vi "test Add and Get Timing Channels.vi"(8 "error in":errorcluster, 11 "TestCase in":refnum<class "Scripting.lvclass">) -> (0 "error out":errorcluster)   [LabVIEW 2024, in "Scripting.lvclass"]
uses:
  Scripting.lvclass
  <vilib>/NI VeriStand/Custom Device API/Custom Device Item Ref.ctl
  Scripting.lvclass/Scripting.ctl
  <vilib>/addons/_JKI Toolkits/VI Tester/TestCase.llb/TestCase.lvclass
  Scripting/AIM/AIM ARINC 429 Scripting.lvlib
  <vilib>/NI VeriStand/Custom Device API/Custom Device API.lvlib
  C:/Program Files/National Instruments/LabVIEW 2024/vi.lib/addons/_JKI Toolkits/VI Tester/TestCase.llb/TestCase.lvclass
panel:
  out "TestCase out":refnum<class "Scripting.lvclass">
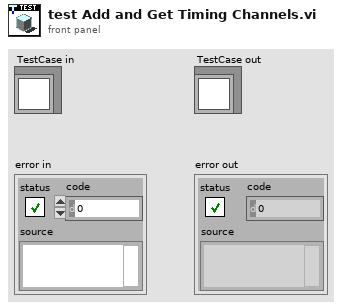
[diagram p1: front panel]
types:
  T1 = typedef "Custom Device API.lvlib/Custom Device Item Ref.ctl" = u64
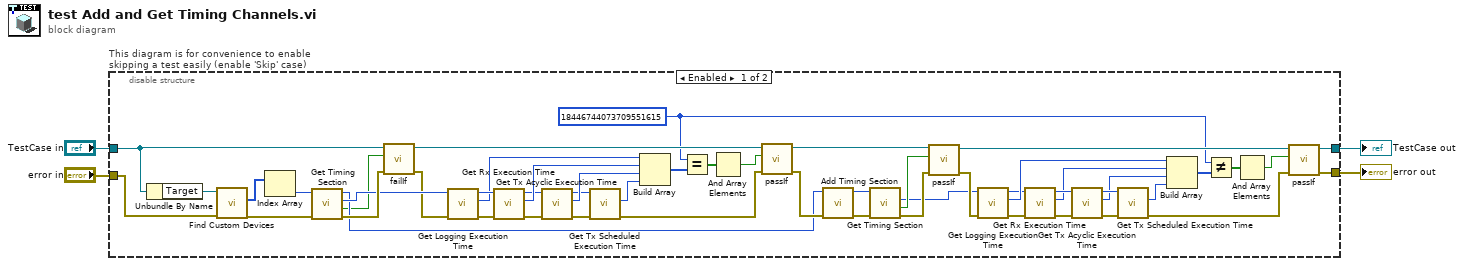
[diagram p0: block diagram]
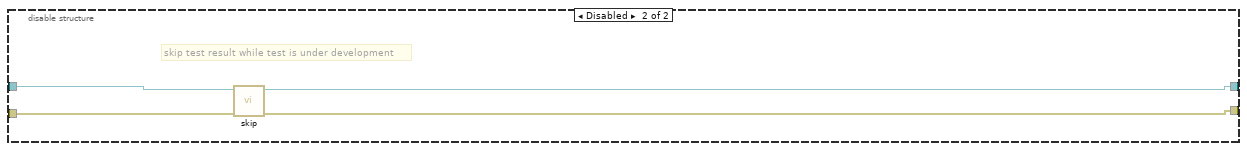
[diagram p2: hidden frame]
diagram:
  n1 = disable-structure "This diagram is for convenience to enable skipping a test easily (enable 'Skip' case)" shown="Enabled" {
    disable-tunnel: "TestCase in" -> [w56 w60]
    disable-tunnel: [w25 w58] -> w1
    disable-tunnel: [w26 w59] -> w3
    disable-tunnel: "error in" -> [w54 w57]
    frame Enabled {
      w5 = T1 18446744073709551615 ("sched tx execution time ref")
      n2 = Unbundle By Name(w56) -> ("Target"=w55:refnum<k24>)
      n3 = call "Find Custom Devices.vi"("error in"=w54, "target"=w55) -> ("error out"=w51:errorcluster, "AIM ARINC 429 custom devices"=w53:T1[])  [unwired: 7 in, 1 out]
      n4 = Index Array(array=w53) -> (element=w52:T1)  [unwired: 1 in]
      n5 = call "Get Timing Section.vi"("error in"=w51, "custom device ref"=w52) -> ("error out"=w50:errorcluster, "Found"=w24:bool, "timing"=w45:T1, "custom device ref out"=w38:T1)  [unwired: 6 in]
      n6 = call-dynamic "failIf.vi"("error in (no error)"=w50, "fail"=w24, "TestCase in"=w56) -> ("error out"=w19:errorcluster, "TestCase out"=w44:refnum<class "Scripting.lvclass">)  [unwired: 7 in]
      n7 = call "Get Logging Execution Time.vi"("error in"=w19, "timing ref"=w45) -> ("error out"=w18:errorcluster, "logging execution time ref"=w17:T1, "timing ref out"=w20:T1)  [unwired: 7 in]
      n8 = call "Get Rx Execution Time.vi"("error in"=w18, "timing ref"=w20) -> ("error out"=w47:errorcluster, "rx execution time ref"=w42:T1, "timing ref out"=w31:T1)  [unwired: 7 in]
      n9 = call "Get Tx Acyclic Execution Time.vi"("error in"=w47, "timing ref"=w31) -> ("error out"=w46:errorcluster, "async tx execution time ref"=w41:T1, "timing ref out"=w30:T1)  [unwired: 7 in]
      n10 = call "Get Tx Scheduled Execution Time.vi"("error in"=w46, "timing ref"=w30) -> ("error out"=w43:errorcluster, "sched tx execution time ref"=w40:T1)  [unwired: 7 in, 1 out]
      n11 = Build Array(w17, w42, w41, w40) -> (w11:T1[])
      n12 = Equal?(x=w5, y=w11) -> (x = y?=w10:bool[])
      n13 = And Array Elements(Boolean array=w10) -> (logical AND=w9:bool)
      n14 = call-dynamic "passIf.vi"("error in (no error)"=w43, "pass"=w9, "TestCase in"=w44) -> ("error out"=w39:errorcluster, "TestCase out"=w37:refnum<class "Scripting.lvclass">)  [unwired: 7 in]
      n15 = call "Add Timing Section.vi"("error in"=w39, "custom device ref"=w38) -> ("error out"=w49:errorcluster, "custom device ref out"=w48:T1)  [unwired: 7 in, 1 out]
      n16 = call "Get Timing Section.vi"("error in"=w49, "custom device ref"=w48) -> ("error out"=w35:errorcluster, "Found"=w23:bool, "timing"=w12:T1)  [unwired: 6 in, 1 out]
      n17 = call-dynamic "passIf.vi"("error in (no error)"=w35, "pass"=w23, "TestCase in"=w37) -> ("error out"=w13:errorcluster, "TestCase out"=w22:refnum<class "Scripting.lvclass">)  [unwired: 7 in]
      n18 = call "Get Logging Execution Time.vi"("error in"=w13, "timing ref"=w12) -> ("error out"=w16:errorcluster, "logging execution time ref"=w15:T1, "timing ref out"=w14:T1)  [unwired: 7 in]
      n19 = call "Get Rx Execution Time.vi"("error in"=w16, "timing ref"=w14) -> ("error out"=w36:errorcluster, "rx execution time ref"=w29:T1, "timing ref out"=w33:T1)  [unwired: 7 in]
      n20 = call "Get Tx Acyclic Execution Time.vi"("error in"=w36, "timing ref"=w33) -> ("error out"=w34:errorcluster, "async tx execution time ref"=w28:T1, "timing ref out"=w32:T1)  [unwired: 7 in]
      n21 = call "Get Tx Scheduled Execution Time.vi"("error in"=w34, "timing ref"=w32) -> ("error out"=w21:errorcluster, "sched tx execution time ref"=w27:T1)  [unwired: 7 in, 1 out]
      n22 = Build Array(w15, w29, w28, w27) -> (w7:T1[])
      n23 = Not Equal?(x=w5, y=w7) -> (x != y?=w8:bool[])
      n24 = And Array Elements(Boolean array=w8) -> (logical AND=w6:bool)
      n25 = call-dynamic "passIf.vi"("error in (no error)"=w21, "pass"=w6, "TestCase in"=w22) -> ("error out"=w26:errorcluster, "TestCase out"=w25:refnum<class "Scripting.lvclass">)  [unwired: 7 in]
    }
    frame Disabled {
      # "skip test result while test is under development"
      n26 = call <vilib>:"skip.vi"("error in (no error)"=w57, "TestCase in"=w60) -> ("error out"=w59:errorcluster, "TestCase out"=w58:refnum<class "Scripting.lvclass">)  [unwired: 8 in]
    }
  }
  "error out" <- w3
  "TestCase out" <- w1
